vi "Save_Op.vi"(4 "Instrument":string, 5 "Surname":string, 6 "Lab":string, 7 "Name":string, 8 "Error In":errorcluster, 10 "Path In":path, 11 "Queue in":refnum<queue>) -> (0 "Error Out":errorcluster, 3 "Path Out":path)   [LabVIEW 2021, in "Main.lvlib" / "Main_Programs_SubVIs.lvlib"]
doc: "This subVI is used for the save operation."
uses:
  Main_Programs_SubVIs.lvlib
  Tipski Definicii/Save_Sostojbi.ctl
  Polymorphic/Enq_Save_QMH.vi
  Signal/Signal.lvlib
  Polymorphic/Queues.lvlib
panel:
  # "Input"
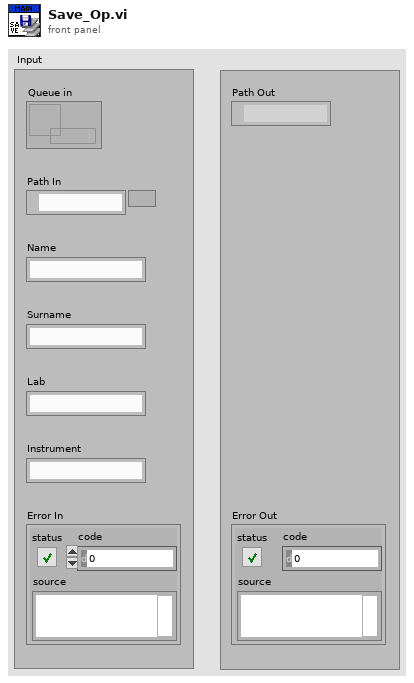
[diagram p1: front panel]
types:
  T1 = enum16{"Check Name", "Check Surname", "Check Lab", "Check Instrument"}
  T2 = typedef "Save_Sostojbi.ctl" = enum16{"Init", "Generate Message", "Pick Path", "Save", "End"}
  T3 = enum16{"Init", "Add String", "Error", "Get Error and Strings", "Reset"}
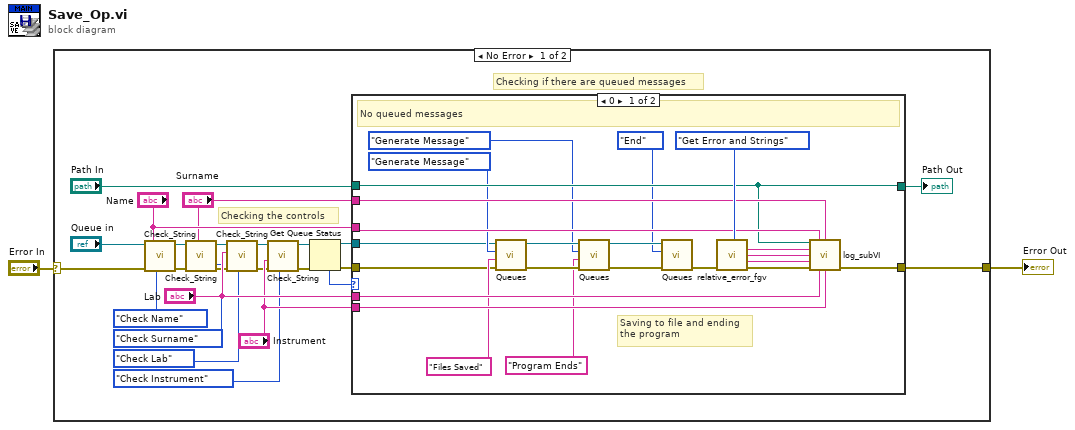
[diagram p0: block diagram]
diagram:
  n1 = case shown="No Error" "Error In" {
    selector: "Error In" -> [w5 w52]
    tunnel: [w26 w52] -> w2
    frame No Error {
      # "Checking the controls"
      # "Checking if there are queued messages"
      n2 = call "Check_String.vi"("Action"=T1."Check Name", "Name"="Name", "Error In"=w5, "Queue In"="Queue in") -> ("Error Out"=w7:errorcluster, "Queue Out"=w9:refnum<queue>)  [unwired: 6 in]
      n3 = call "Check_String.vi"("Surname"="Surname", "Action"=T1."Check Surname", "Error In"=w7, "Queue In"=w9) -> ("Error Out"=w11:errorcluster, "Queue Out"=w12:refnum<queue>)  [unwired: 6 in]
      n4 = call "Check_String.vi"("Action"=T1."Check Lab", "Error In"=w11, "Lab"="Lab", "Queue In"=w12) -> ("Error Out"=w14:errorcluster, "Queue Out"=w15:refnum<queue>)  [unwired: 6 in]
      n5 = call "Check_String.vi"("Action"=T1."Check Instrument", "Error In"=w14, "Instrument"="Instrument", "Queue In"=w15) -> ("Error Out"=w17:errorcluster, "Queue Out"=w18:refnum<queue>)  [unwired: 6 in]
      n6 = Get Queue Status(queue=w18, error in (no error)=w17) -> (queue out=w21:refnum<queue>, error out=w20:errorcluster, # elements in queue=w19:i32)  [unwired: 1 in, 5 out]
      n7 = case shown="0" w19 {
        tunnel: w20 -> [w28 w51]
        tunnel: w21 -> [w29 _]
        tunnel: "Instrument" -> [w44 _]
        tunnel: "Lab" -> [w43 _]
        tunnel: "Surname" -> [w42 _]
        tunnel: "Name" -> [w41 _]
        tunnel: [w40 w51] -> w26
        tunnel: "Path In" -> [w39 w50]
        tunnel: [w39 w50] -> w3
        frame 0 {
          # "Saving to file and ending\nthe program"
          # "No queued messages"
          n8 = call-poly "Queues.vi"("Error In"=w28, "Message"="Files Saved", "Instruction"=Save_Sostojbi."Generate Message", "Queue In"=w29) -> ("Error Out"=w36:errorcluster, "Queue Out"=w35:refnum<queue>)  [unwired: 6 in]
          n9 = call-poly "Queues.vi"("Error In"=w36, "Message"="Program Ends", "Instruction"=Save_Sostojbi."Generate Message", "Queue In"=w35) -> ("Error Out"=w32:errorcluster, "Queue Out"=w31:refnum<queue>)  [unwired: 6 in]
          n10 = call-poly "Queues.vi"("Error In"=w32, "Instruction"=Save_Sostojbi."End", "Queue In"=w31) -> ("Error Out"=w27:errorcluster)  [unwired: 7 in, 1 out]
          n11 = call "relative_error_fgv.vi"("Error In"=w27, "Action"=T3."Get Error and Strings") -> ("Error Out"=w49:errorcluster, "Error String"=w47:string, "Incremented String"=w46:string, "Starting String"=w45:string)  [unwired: 5 in, 1 out]
          n12 = call "log_subVI.vi"("Path"=w39, "Name"=w41, "Surname"=w42, "True Value"=w45, "Incremented"=w46, "Error"=w47, "Error In"=w49, "Lab"=w43, "Instrument"=w44) -> ("Error Out"=w40:errorcluster)  [unwired: 6 in]
        }
        frame 1, Default {
          # "Means that some inputs are empty"
          # "There are queued messages"
        }
      }
      "Path Out" <- w3
    }
    frame Error {
    }
  }
  "Error Out" <- w2
